vi "Open Butterfly Drive.vi"(8 "error in (no error)":errorcluster, 9 "secondsFromNeutralToFull":dbl, 10 "Brake/Coast":enum16{"Coast", "Brake"}(ring)=enum."Brake", 11 "Cluster":T1) -> (0 "error out":errorcluster)   [LabVIEW 2018]
uses:
  <vilib>/Rock Robotics/WPI/SafetyOutput/WPI_SafetyOutputConfigMenu.ctl
  <vilib>/Rock Robotics/WPI/ThirdParty/Phoenix-LabVIEW/Motor Controller/Controls/CTRE_Phoenix_MotorControl_NeutralMode.ctl
  <vilib>/Rock Robotics/WPI/RobotDrive/WPI_RobotDriveOpen2MotorWithExistingMotors.vi
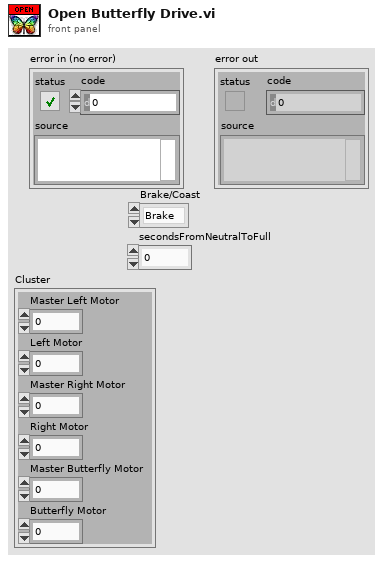
[diagram p1: front panel]
types:
  T1 = cluster{"Master Left Motor":u8, "Left Motor":u8, "Master Right Motor":u8, "Right Motor":u8, "Master Butterfly Motor":i32, "Butterfly Motor":i32}
  T2 = enum16{"FollowerType_PercentOutput", "FollowerType_AuxOutput1"}
  T3 = typedef "CTRE_Phoenix_MotorControl_NeutralMode.ctl" = enum8{"EEPROMSetting", "Override to Coast", "Override to Brake"}
  T4 = typedef "WPI_SafetyOutputConfigMenu.ctl" = enum16{"Enable", "Disable"}
  T5 = typedef "WPI_MotorControlDeviceRef.ctl" = cluster{"DeviceStatus":errorcluster, "Type":T6, "PWM":cluster{"PWM Channel":T7, "DeadBand":T8}, "CAN":cluster{"Device Number":u8, "SetOutput VI Ref":variant, "GetOutput VI Ref":variant, "Enable VI Ref":variant, "Disable VI Ref":variant, "Data":variant}, "Invert":bool, "DIO PWM":cluster{"PWM \"Enable\" Channel":T7, "DIOChannel":T9, "PWM Rate":dbl}}
  T6 = typedef "WPI_MotorControlType.ctl" = enum16{"PWM", "CAN", "DIO PWM"}
  T7 = typedef "FPGA_DIOPWMChannel.ctl" = enum8{"PWM 0", "PWM 1", "PWM 2", "PWM 3", "PWM 4", "PWM 5", "PWM 6", "PWM 7", "PWM 8", "PWM 9", "PWM MXP 0", "PWM MXP 1", "PWM MXP 2", "PWM MXP 3", "PWM MXP 4", "PWM MXP 5", "PWM MXP 6", "PWM MXP 7", "PWM MXP 8", "PWM MXP 9", "Invalid"}
  T8 = typedef "WPI_PWMDeadband.ctl" = cluster{"Name":string, "maxPositivePwm":i32, "minPositivePwm":i32, "centerPwm":i32, "maxNegativePwm":i32, "minNegativePwm":i32, "angularRange":u16}
  T9 = typedef "FPGA_DIOChannel.ctl" = enum8{"DIO 0", "DIO 1", "DIO 2", "DIO 3", "DIO 4", "DIO 5", "DIO 6", "DIO 7", "DIO 8", "DIO 9", "DIO MXP 0", "DIO MXP 1", "DIO MXP 2", "DIO MXP 3", "DIO MXP 4", "DIO MXP 5", "DIO MXP 6", "DIO MXP 7", "DIO MXP 8", "DIO MXP 9", "DIO MXP 10", "DIO MXP 11", "DIO MXP 12", "DIO MXP 13", "DIO MXP 14", "DIO MXP 15", "SPI Port CS1", "SPI Port CS2", "SPI Port CS3", "SPI Port MISO", "SPI Port MOSI", "Invalid"}
  T10 = typedef "WPI_RobotDriveDevRef.ctl" = cluster{"DevStatus":errorcluster, "Motors[]":T5[], "Square Inputs":bool, "Max Output":dbl}
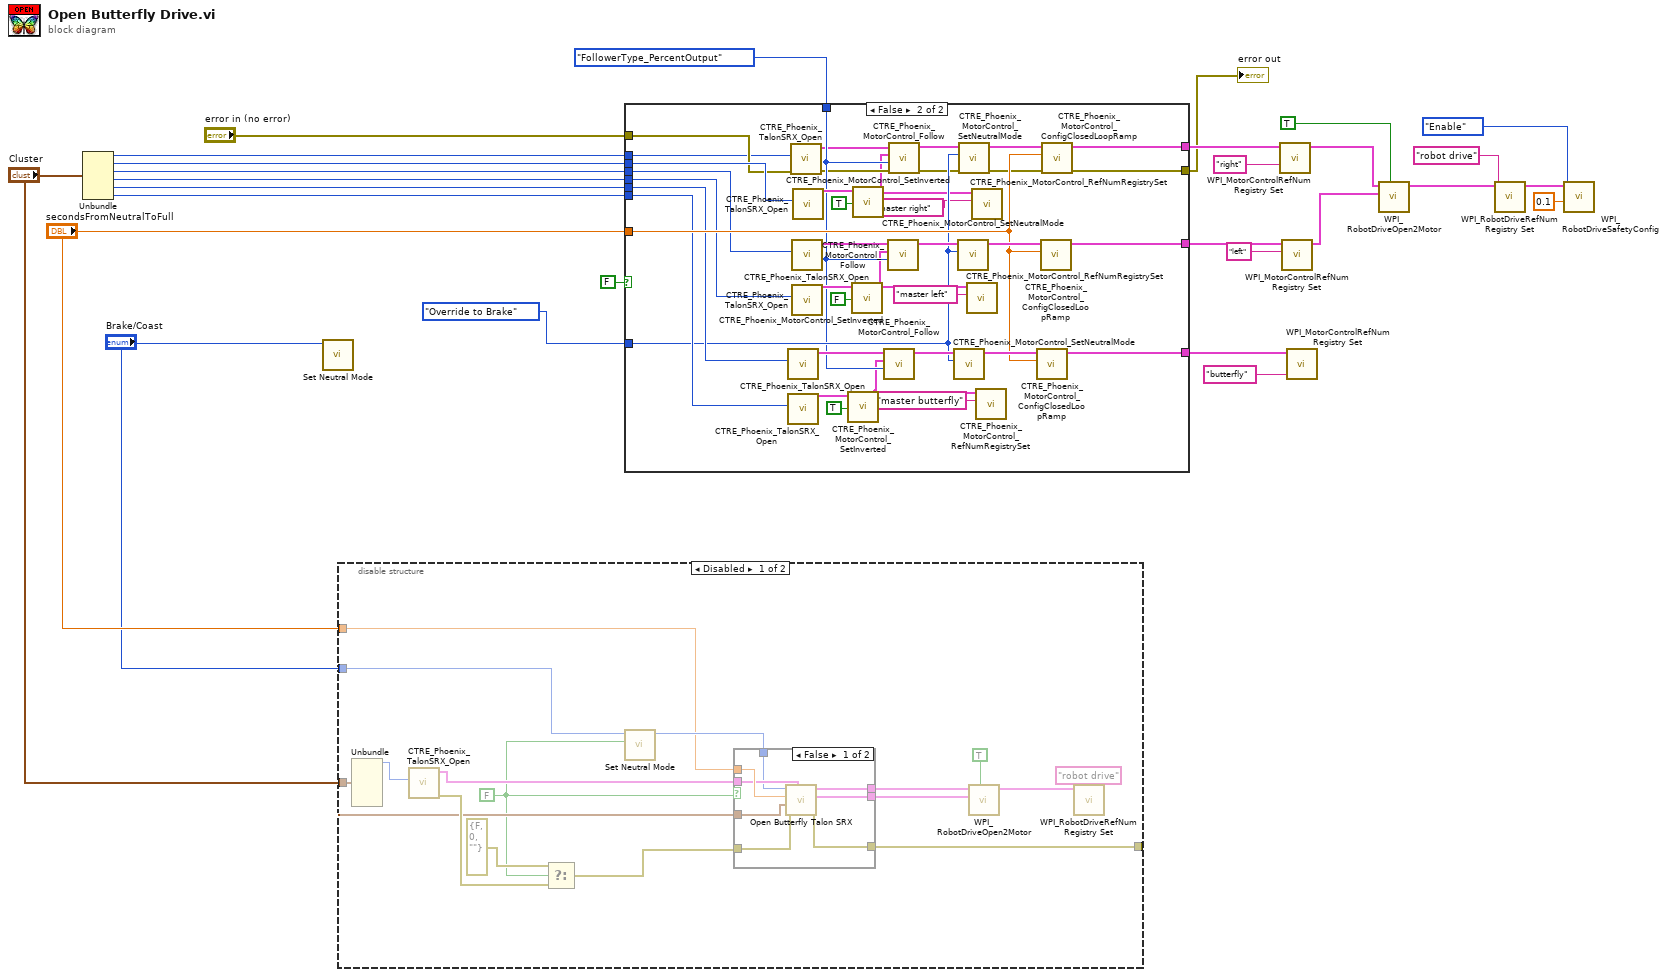
[diagram p0: block diagram]
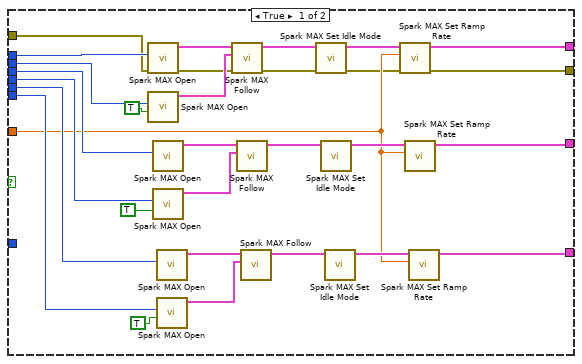
[diagram p2: hidden frame]
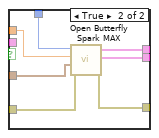
[diagram p3: hidden frame]
diagram:
  n1 = Unbundle("Cluster") -> ("Master Left Motor"=w7:u8, "Left Motor"=w28:u8, "Master Right Motor"=w27:u8, "Right Motor"=w26:u8, "Master Butterfly Motor"=w25:i32, "Butterfly Motor"=w24:i32)
  n2 = call "Set Neutral Mode.vi"("Enum"="Brake/Coast") -> ()  [unwired: 10 in, 1 out]
  n3 = disable-structure shown="Disabled" {
    disable-tunnel: "Brake/Coast" -> [w44 _]
    disable-tunnel: "secondsFromNeutralToFull" -> [w42 _]
    disable-tunnel: [w41 _] -> _
    disable-tunnel: "Cluster" -> [w30 _]
    frame Disabled {
      w29 = FALSE
      n4 = Unbundle(w30) -> ("Master Left Motor"=w43:u8)  [unwired: 5 out]
      n5 = call <vilib>:"CTRE_Phoenix_TalonSRX_Open.vi"("Device Number"=w43) -> ("error out"=w37:errorcluster, "CAN Talon SRX Ref"=w35:T5, "error in"=w36:errorcluster)  [unwired: 8 in]
      n6 = Select(t=errorcluster {"status"=FALSE, "code"=0, "source"=""} ("error out"), s=w29, f=w37) -> (s? t:f=w40:errorcluster)
      n7 = call "Set Neutral Mode.vi"("status"=w29, "Enum"=w44) -> ("Motor Control Neutral Mode"=w45:u16)  [unwired: 9 in]
      n8 = case shown="False" w29 {
        tunnel: [w53 w60] -> w34
        tunnel: w35 -> [w48 _]
        tunnel: [w52 w59] -> w39
        tunnel: w40 -> [w51 w58]
        tunnel: [w50 w57] -> w41
        tunnel: w42 -> [w49 w56]
        tunnel: w30 -> [w46 w54]
        tunnel: w45 -> [w47 w55]
        frame False {
          n9 = call "Open Butterfly Talon SRX.vi"("CAN Talon SRX Ref"=w48, "error in (no error)"=w51, "Cluster"=w46, "secondsFromNeutralToFull"=w49, "Motor Control Neutral Mode"=w47) -> ("error out"=w50:errorcluster, "PhoenixMotorControlDevRef"=w52:T5, "PhoenixMotorControlDevRef 2"=w53:T5)  [unwired: 4 in]
        }
        frame True {
          n10 = call "Open Butterfly Spark MAX.vi"("error in (no error)"=w58, "Cluster"=w54, "Seconds from neutral to full (0)"=w56, "Idle Mode"=w55) -> ("error out"=w57:errorcluster, "right drive"=w59:T5, "left drive"=w60:T5)  [unwired: 4 in, 1 out]
        }
      }
      n11 = call-poly <vilib>:"WPI_RobotDriveOpen2Motor.vi"("Square Inputs"=TRUE, "Right Motor Dev Ref"=w39, "Left Motor Dev Ref"=w34) -> ("RobotDriveDevRef"=w32:T10)  [unwired: 7 in, 1 out]
      n12 = call <vilib>:"WPI_RobotDriveRefNum Registry Set.vi"("refnum name"="robot drive", "RobotDriveDevRef"=w32) -> ()  [unwired: 8 in, 2 out]
    }
    frame Enabled {
    }
  }
  n13 = case shown="False" FALSE {
    tunnel: "secondsFromNeutralToFull" -> [w69 w114]
    tunnel: w7 -> [w77 w97]
    tunnel: w28 -> [w76 w113]
    tunnel: w27 -> [w75 w112]
    tunnel: w26 -> [w74 w111]
    tunnel: w25 -> [w73 w110]
    tunnel: w24 -> [w70 w109]
    tunnel: CTRE_Phoenix_MotorControl_NeutralMode."Override to Brake" ("Motor Control Neutral Mode") -> [_ w108]
    tunnel: [w68 w107] -> w23
    tunnel: [w67 w106] -> w22
    tunnel: [w66 w105] -> w21
    tunnel: "error in (no error)" -> [w65 w98]
    tunnel: [w61 w102] -> w5
    tunnel: T2."FollowerType_PercentOutput" ("FollowerType") -> [_ w101]
    frame True {
      n14 = call <vilib>:"Spark MAX Open.vi"("error in (no error)"=w65, "Device Number"=w77) -> ("error out"=w64:errorcluster, "MotorControlDeviceRef"=w87:T5)  [unwired: 8 in]
      n15 = call <vilib>:"Spark MAX Open.vi"("Invert"=TRUE, "Device Number"=w76) -> ("MotorControlDeviceRef"=w88:T5)  [unwired: 8 in, 1 out]
      n16 = call <vilib>:"Spark MAX Open.vi"("Device Number"=w75) -> ("MotorControlDeviceRef"=w85:T5)  [unwired: 9 in, 1 out]
      n17 = call <vilib>:"Spark MAX Open.vi"("Invert"=TRUE, "Device Number"=w74) -> ("MotorControlDeviceRef"=w84:T5)  [unwired: 8 in, 1 out]
      n18 = call <vilib>:"Spark MAX Open.vi"("Device Number"=w73) -> ("MotorControlDeviceRef"=w78:T5)  [unwired: 9 in, 1 out]
      n19 = call <vilib>:"Spark MAX Open.vi"("Invert"=TRUE, "Device Number"=w70) -> ("MotorControlDeviceRef"=w79:T5)  [unwired: 8 in, 1 out]
      n20 = call <vilib>:"Spark MAX Follow.vi"("error in (no error)"=w64, "Master Controller"=w88, "MotorControlDeviceRef"=w87) -> ("error out"=w63:errorcluster, "MotorControlDeviceRef"=w89:T5)  [unwired: 7 in]
      n21 = call <vilib>:"Spark MAX Follow.vi"("Master Controller"=w84, "MotorControlDeviceRef"=w85) -> ("MotorControlDeviceRef"=w83:T5)  [unwired: 8 in, 1 out]
      n22 = call <vilib>:"Spark MAX Follow.vi"("Master Controller"=w79, "MotorControlDeviceRef"=w78) -> ("MotorControlDeviceRef"=w80:T5)  [unwired: 8 in, 1 out]
      n23 = call <vilib>:"Spark MAX Set Idle Mode.vi"("error in (no error)"=w63, "MotorControlDeviceRef in"=w89) -> ("error out"=w62:errorcluster, "MotorControlDeviceRef out"=w90:T5)  [unwired: 8 in]
      n24 = call <vilib>:"Spark MAX Set Idle Mode.vi"("MotorControlDeviceRef in"=w83) -> ("MotorControlDeviceRef out"=w82:T5)  [unwired: 9 in, 1 out]
      n25 = call <vilib>:"Spark MAX Set Idle Mode.vi"("MotorControlDeviceRef in"=w80) -> ("MotorControlDeviceRef out"=w81:T5)  [unwired: 9 in, 1 out]
      n26 = call <vilib>:"Spark MAX Set Ramp Rate.vi"("error in (no error)"=w62, "Seconds from neutral to full (0)"=w69, "MotorControlDeviceRef in"=w90) -> ("error out"=w61:errorcluster, "MotorControlDeviceRef"=w68:T5)  [unwired: 7 in]
      n27 = call <vilib>:"Spark MAX Set Ramp Rate.vi"("Seconds from neutral to full (0)"=w69, "MotorControlDeviceRef in"=w82) -> ("MotorControlDeviceRef"=w67:T5)  [unwired: 8 in, 1 out]
      n28 = call <vilib>:"Spark MAX Set Ramp Rate.vi"("Seconds from neutral to full (0)"=w69, "MotorControlDeviceRef in"=w81) -> ("MotorControlDeviceRef"=w66:T5)  [unwired: 8 in, 1 out]
    }
    frame False {
      n29 = call <vilib>:"CTRE_Phoenix_TalonSRX_Open.vi"("Device Number"=w110) -> ("CAN Talon SRX Ref"=w119:T5)  [unwired: 9 in, 1 out]
      n30 = call <vilib>:"CTRE_Phoenix_TalonSRX_Open.vi"("Device Number"=w109) -> ("CAN Talon SRX Ref"=w118:T5)  [unwired: 9 in, 1 out]
      n31 = call <vilib>:"CTRE_Phoenix_TalonSRX_Open.vi"("error in"=w98, "Device Number"=w97) -> ("error out"=w99:errorcluster, "CAN Talon SRX Ref"=w100:T5)  [unwired: 8 in]
      n32 = call <vilib>:"CTRE_Phoenix_TalonSRX_Open.vi"("Device Number"=w112) -> ("CAN Talon SRX Ref"=w120:T5)  [unwired: 9 in, 1 out]
      n33 = call <vilib>:"CTRE_Phoenix_TalonSRX_Open.vi"("Device Number"=w111) -> ("CAN Talon SRX Ref"=w121:T5)  [unwired: 9 in, 1 out]
      n34 = call <vilib>:"CTRE_Phoenix_TalonSRX_Open.vi"("Device Number"=w113) -> ("CAN Talon SRX Ref"=w128:T5)  [unwired: 9 in, 1 out]
      n35 = call <vilib>:"CTRE_Phoenix_MotorControl_SetInverted.vi"("Invert?"=TRUE, "PhoenixMotorControlDevRef"=w118) -> ("PhoenixMotorControlDevRef"=w94:T5)  [unwired: 8 in, 1 out]
      n36 = call <vilib>:"CTRE_Phoenix_MotorControl_SetInverted.vi"("Invert?"=FALSE, "PhoenixMotorControlDevRef"=w121) -> ("PhoenixMotorControlDevRef"=w96:T5)  [unwired: 8 in, 1 out]
      n37 = call <vilib>:"CTRE_Phoenix_MotorControl_SetInverted.vi"("Invert?"=TRUE, "PhoenixMotorControlDevRef"=w128) -> ("PhoenixMotorControlDevRef"=w95:T5)  [unwired: 8 in, 1 out]
      n38 = call <vilib>:"CTRE_Phoenix_MotorControl_Follow.vi"("FollowerType"=w101, "Master Controller to Follow"=w94, "PhoenixMotorControlDevRef"=w119) -> ("PhoenixMotorControlDevRef"=w116:T5)  [unwired: 7 in, 1 out]
      n39 = call <vilib>:"CTRE_Phoenix_MotorControl_Follow.vi"("FollowerType"=w101, "Master Controller to Follow"=w96, "PhoenixMotorControlDevRef"=w120) -> ("PhoenixMotorControlDevRef"=w123:T5)  [unwired: 7 in, 1 out]
      n40 = call <vilib>:"CTRE_Phoenix_MotorControl_Follow.vi"("error in (no error)"=w99, "FollowerType"=w101, "Master Controller to Follow"=w95, "PhoenixMotorControlDevRef"=w100) -> ("error out"=w104:errorcluster, "PhoenixMotorControlDevRef"=w126:T5)  [unwired: 6 in]
      n41 = call <vilib>:"CTRE_Phoenix_MotorControl_SetNeutralMode.vi"("Motor Control Neutral Mode"=w108, "PhoenixMotorControlDevRef"=w116) -> ("PhoenixMotorControlDevRef"=w115:T5)  [unwired: 8 in, 1 out]
      n42 = call <vilib>:"CTRE_Phoenix_MotorControl_SetNeutralMode.vi"("Motor Control Neutral Mode"=w108, "PhoenixMotorControlDevRef"=w123) -> ("PhoenixMotorControlDevRef"=w124:T5)  [unwired: 8 in, 1 out]
      n43 = call <vilib>:"CTRE_Phoenix_MotorControl_SetNeutralMode.vi"("error in (no error)"=w104, "Motor Control Neutral Mode"=w108, "PhoenixMotorControlDevRef"=w126) -> ("error out"=w103:errorcluster, "PhoenixMotorControlDevRef"=w125:T5)  [unwired: 7 in]
      n44 = call <vilib>:"CTRE_Phoenix_MotorControl_RefNumRegistrySet.vi"("refnum name"="master left", "PhoenixMotorControlDevRef"=w96) -> ()  [unwired: 8 in, 2 out]
      n45 = call <vilib>:"CTRE_Phoenix_MotorControl_RefNumRegistrySet.vi"("refnum name"="master right", "PhoenixMotorControlDevRef"=w95) -> ()  [unwired: 8 in, 2 out]
      n46 = call <vilib>:"CTRE_Phoenix_MotorControl_RefNumRegistrySet.vi"("refnum name"="master butterfly", "PhoenixMotorControlDevRef"=w94) -> ()  [unwired: 8 in, 2 out]
      n47 = call <vilib>:"CTRE_Phoenix_MotorControl_ConfigClosedLoopRamp.vi"("secondsFromNeutralToFull"=w114, "PhoenixMotorControlDevRef"=w115) -> ("PhoenixMotorControlDevRef"=w105:T5)  [unwired: 8 in, 1 out]
      n48 = call <vilib>:"CTRE_Phoenix_MotorControl_ConfigClosedLoopRamp.vi"("secondsFromNeutralToFull"=w114, "PhoenixMotorControlDevRef"=w124) -> ("PhoenixMotorControlDevRef"=w106:T5)  [unwired: 8 in, 1 out]
      n49 = call <vilib>:"CTRE_Phoenix_MotorControl_ConfigClosedLoopRamp.vi"("error in (no error)"=w103, "secondsFromNeutralToFull"=w114, "PhoenixMotorControlDevRef"=w125) -> ("error out"=w102:errorcluster, "PhoenixMotorControlDevRef"=w107:T5)  [unwired: 7 in]
    }
  }
  "error out" <- w5
  n50 = call <vilib>:"WPI_MotorControlRefNum Registry Set.vi"("refnum name"="right", "MotorControlDevRef"=w23) -> ("MotorControlDevRef"=w17:T5)  [unwired: 8 in, 1 out]
  n51 = call <vilib>:"WPI_MotorControlRefNum Registry Set.vi"("refnum name"="left", "MotorControlDevRef"=w22) -> ("MotorControlDevRef"=w16:T5)  [unwired: 8 in, 1 out]
  n52 = call <vilib>:"WPI_MotorControlRefNum Registry Set.vi"("refnum name"="butterfly", "MotorControlDevRef"=w21) -> ()  [unwired: 8 in, 2 out]
  n53 = call-poly <vilib>:"WPI_RobotDriveOpen2Motor.vi"("Square Inputs"=TRUE, "Right Motor Dev Ref"=w16, "Left Motor Dev Ref"=w17) -> ("RobotDriveDevRef"=w14:T10)  [unwired: 7 in, 1 out]
  n54 = call <vilib>:"WPI_RobotDriveRefNum Registry Set.vi"("refnum name"="robot drive", "RobotDriveDevRef"=w14) -> ("RobotDriveDevRef"=w12:T10)  [unwired: 8 in, 1 out]
  n55 = call <vilib>:"WPI_RobotDriveSafetyConfig.vi"("timeout (s)"=0.1, "mode"=WPI_SafetyOutputConfigMenu."Enable", "RobotDriveDevRef"=w12) -> ()  [unwired: 7 in, 2 out]
